vi "test Container ACL.vi"(8 "error in (no error)":errorcluster, 11 "TestCase in":refnum<class "Test_Blob.lvclass">) -> (0 "error out":errorcluster, 3 "TestCase out":refnum<class "Test_Blob.lvclass">)   [LabVIEW 2015, in "Test_Blob.lvclass"]
uses:
  Test_Blob.lvclass
  Blob Storage/Signed Identifier.ctl
  Blob Storage/Access Policy.ctl
  Global Parameters.vi
  Core/Session/Session.lvclass
  Blob Storage/NI_Azure_Blob.lvlib
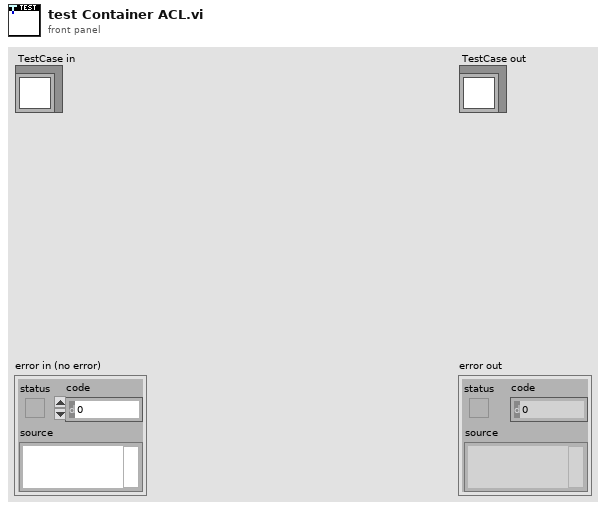
[diagram p1: front panel]
types:
  T1 = typedef "NI_Azure_Blob.lvlib/Signed Identifier.ctl" = cluster{"ID":string, "Access policy":T2}
  T2 = typedef "NI_Azure_Blob.lvlib/Access Policy.ctl" = cluster{"Start":string, "Expiry":string, "Permission":string}
  T3 = typedef "NI_Azure_Core.lvlib/Session.lvclass/Azure Credentials.ctl" = cluster{"Storage Account Name":string, "Access Key":string}
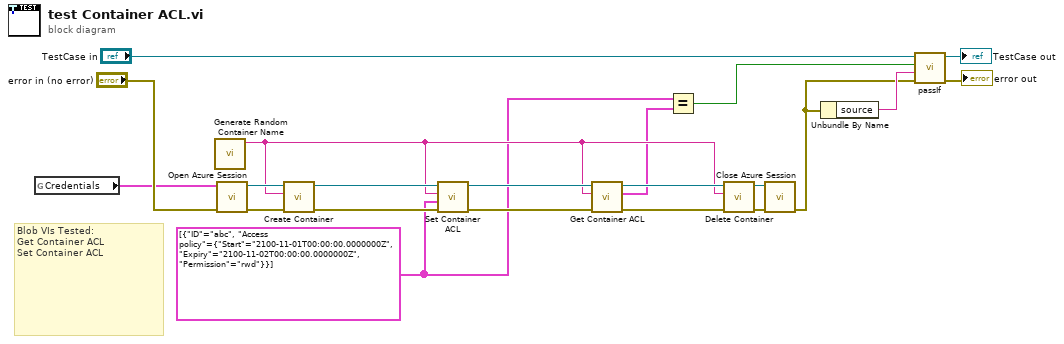
[diagram p0: block diagram]
diagram:
  w1 = T1[] [{"ID"="abc", "Access policy"={"Start"="2100-11-01T00:00:00.0000000Z", "Expiry"="2100-11-02T00:00:00.0000000Z", "Permission"="rwd"}}] ("ACL")
  # "Blob VIs Tested:\nGet Container ACL\nSet Container ACL"
  n1 = global read "Global Parameters.vi" "Credentials"() -> (w14:T3)
  n2 = call "Generate Random Container Name.vi"() -> ("Random Container Name"=w4:string)  [unwired: 11 in]
  n3 = call "Open Azure Session.vi"("error in (no error)"="error in (no error)", "Credentials"=w14) -> ("error out"=w15:errorcluster, "Azure Session"=w12:refnum<class "Session.lvclass">)  [unwired: 8 in]
  n4 = call "Create Container.vi"("error in (no error)"=w15, "Container"=w4, "Azure Session in"=w12) -> ("error out"=w17:errorcluster, "Azure Session out"=w6:refnum<class "Session.lvclass">)  [unwired: 7 in]
  n5 = call "Set Container ACL.vi"("error in (no error)"=w17, "ACL"=w1, "Container"=w4, "Azure Session in"=w6) -> ("error out"=w7:errorcluster, "Azure Session out"=w5:refnum<class "Session.lvclass">)  [unwired: 6 in]
  n6 = call "Get Container ACL.vi"("error in (no error)"=w7, "Container"=w4, "Azure Session in"=w5) -> ("error out"=w9:errorcluster, "ACL"=w2:T1[], "Azure Session out"=w8:refnum<class "Session.lvclass">)  [unwired: 6 in]
  n7 = Equal?(x=w1, y=w2) -> (x = y?=w3:bool)
  n8 = call "Delete Container.vi"("error in (no error)"=w9, "Container"=w4, "Azure Session in"=w8) -> ("error out"=w13:errorcluster, "Azure Session out"=w11:refnum<class "Session.lvclass">)  [unwired: 7 in]
  n9 = call "Close Azure Session.vi"("error in (no error)"=w13, "Azure Session"=w11) -> ("error out"=w10:errorcluster)  [unwired: 9 in]
  n10 = Unbundle By Name(w10) -> ("source"=w18:string)
  n11 = call-dynamic "passIf.vi"("error in (no error)"=w10, "message (\"\")"=w18, "pass"=w3, "TestCase in"="TestCase in") -> ("error out"=→"error out":errorcluster, "TestCase out"=→"TestCase out":refnum<class "Test_Blob.lvclass">)  [unwired: 6 in]
